vi "myRIO_BRig_RT_dataCurrent_idxDataLick.vi"() -> (2 "output_idxDataLick":i32)   [LabVIEW 2014]
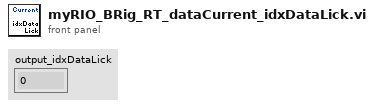
[diagram p1: front panel]
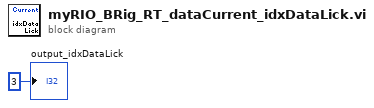
[diagram p0: block diagram]
diagram:
  "output_idxDataLick" <- 3 ("output_iBlock")
